vi "DrawHud.vi"(8 "error in (no error)":errorcluster, 10 "Font":string="content/fonts/neuropol.ttf", 11 "Player in":refnum<class "Player.lvclass">) -> (0 "error out":errorcluster, 3 "Player out":refnum<class "Player.lvclass">)   [LabVIEW 2015, in "Player.lvclass"]
uses:
  Player.lvclass
  Player.lvclass/Player.ctl
  3D Object/3D Object.lvclass/3D Object.ctl
  <vilib>/picture/3D Picture Control/Transformations/Get Translation.vi
  3D Object/3D Object.lvclass
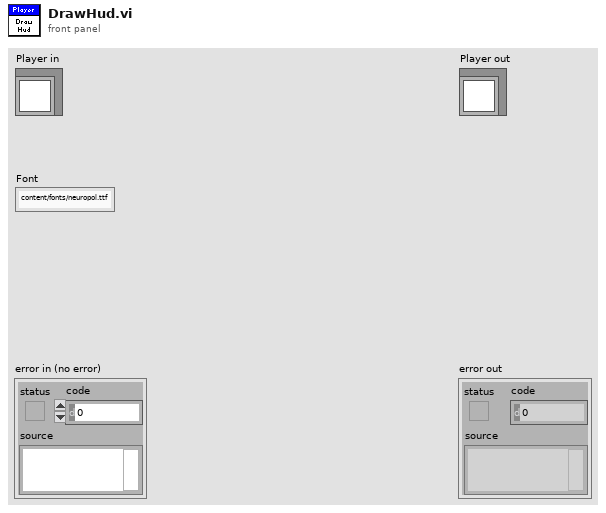
[diagram p1: front panel]
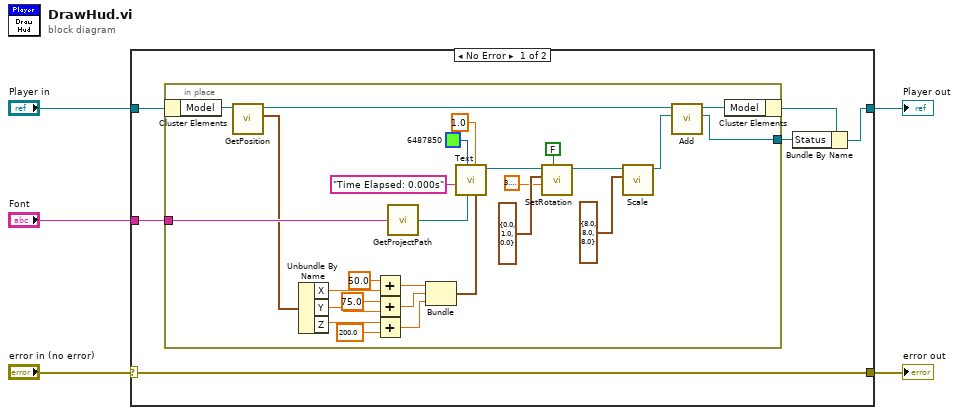
[diagram p0: block diagram]
diagram:
  n1 = case shown="No Error" "error in (no error)" {
    selector: "error in (no error)" -> [w11 w40]
    tunnel: [w11 w40] -> w4
    tunnel: [w7 w39] -> w2
    tunnel: "Player in" -> [w10 w39]
    tunnel: "Font" -> [w9 _]
    frame No Error {
      n2 = in-place {
        in-place-border: w9 -> [w36]
        in-place-border: [w35] -> w6
        n3 = in-place-cluster #1(w10) -> ("Model"=w37:refnum<class "3D Object.lvclass">)
        n4 = call "GetPosition.vi"("3D Object in"=w37) -> ("Position"=w12:cluster{"X":sgl, "Y":sgl, "Z":sgl}, "3D Object out"=w13:refnum<class "3D Object.lvclass">)  [unwired: 8 in, 1 out]
        n5 = Unbundle By Name(w12) -> ("X"=w34:sgl, "Y"=w16:sgl, "Z"=w31:sgl)
        n6 = Add(x=sgl 50.0, y=w34) -> (x+y=w33:sgl)
        n7 = Add(x=sgl 75.0, y=w16) -> (x+y=w17:sgl)
        n8 = Add(x=w31, y=sgl 200.0) -> (x+y=w32:sgl)
        n9 = call "GetProjectPath.vi"("File"=w36) -> ("Path"=w28:path)
        n10 = Bundle(w33, w17, w32) -> (w29:cluster{sgl, sgl, sgl})  [unwired: 1 in]
        n11 = call "Text.vi"("Position"=w29, "Alpha"=1.0, "Path to font file"=w28, "Color Box"=u32 6487850, "Text"="Time Elapsed: 0.000s") -> ("3D Object out"=w25:refnum<class "3D Object.lvclass">)  [unwired: 5 in, 1 out]
        n12 = call "SetRotation.vi"("Relative?"=FALSE, "Angle"=3.141592653589793, "Axis"=cluster{"X":sgl, "Y":sgl, "Z":sgl} {"X"=0.0, "Y"=1.0, "Z"=0.0}, "3D Object in"=w25) -> ("3D Object out"=w21:refnum<class "3D Object.lvclass">)  [unwired: 6 in, 1 out]
        n13 = call "Scale.vi"("Scale"=cluster{"X":sgl, "Y":sgl, "Z":sgl} {"X"=8.0, "Y"=8.0, "Z"=8.0}, "3D Object in"=w21) -> ("3D Object out"=w19:refnum<class "3D Object.lvclass">)  [unwired: 8 in, 1 out]
        n14 = call "Add.vi"("Child in"=w19, "Parent in"=w13) -> ("Child out"=w35:refnum<class "3D Object.lvclass">, "Parent out"=w38:refnum<class "3D Object.lvclass">)  [unwired: 7 in, 1 out]
        n15 = in-place-cluster #1("Model"=w38) -> (w8:refnum<class "Player.lvclass">)
      }
      n16 = Bundle By Name(cluster=w8, "Status"=w6) -> (w7:refnum<class "Player.lvclass">)
    }
    frame Error {
    }
  }
  "error out" <- w4
  "Player out" <- w2
